vi "GetNI_SynthFocus_25.vi"(0 "Digitizer Settings":T4={"Digitizer delay (us) "=0.0, "rf points per line"=2048, "lines per plane"=128, "Samp Rate (Hz)"=100000000.0, "Additional dig delay (us)"=0.0, "Voltage Scale"=0.4, "Pre-Looks"=0, "Offset delay (us)"=0.0, "bits A/D"=8, "Avg Num"=1, "DigTimeOut"=5.0, "Rel Dig Delay"=0.0, "Dig Ch"=0, "LeCroyCluster"={"LeCroy Channels"=[TRUE, FALSE, FALSE, FALSE], "LC read pt offset"=0.0, "Sweep Avg"=FALSE}, "Main Digitizer"=enum."NI Digitizer", "Dig Config"=enum."Single channel", "Digitizer ID Cluster"={"Acqiris/Alazar/SP ID"=[], "NI Instr Handles"=[], "LeCroy VISA"="", "GaGe Handle"={"Handle"=0, "Sample size"=0, "Resolution"=0, "Offset"=0, "Channels"=0, "Boards"=0}, "ATS Ref"="ATS9350", "Acqiris Address"=["PCI::INSTR0"], "ADQRef"=refnum, "adq_cu_ptr"=refnum}, "Trigger Settings"={"Trig Source"=1, "Trig Coupling"=0, "Trig Slope"=0, "Level (mV)"=1500.0}, "Bulk Acq"=FALSE, "Bulk Start Indexes"=[], "Data Ref RF"=refnum, "NI ID/Channel"=[], "Total Dig CH"=1, "Xtra Ann Trig delay (us)"=10.0, "Fix Z Delay?"=FALSE, "One Way Transmission?"=FALSE, "Data Ref Log"=refnum} {"Trigger Settings"."Trig Slope" items=["Positive", "Negative"]; "Trigger Settings"."Level (mV)" format="%.2f"; "Trigger Settings"."Trig Coupling" items=["DC 1 MOhm", "AC 1 MOhm", "DC 50 Ohm", "AC 50 Ohm"]; "Trigger Settings"."Trig Source" items=["Chan 1", "External"]; "Rel Dig Delay" format="%.2f"; "DigTimeOut" format="%.2f"; "Avg Num" min=1; "Offset delay (us)" format="%.2f"; "Additional dig delay (us)" format="%.2f"; "Digitizer delay (us)" format="%.2f"}, 7 "errorin":errorcluster, 8 "File Array":string[](array[string]), 9 "Ann Array Params":T1={"Synth Foc?"=FALSE, "Focal Zones"=41, "Switch T/R"=0, "Trans Geometry (mm)"={"Transducer"=0, "Geo Focus"=12.0, "a (radius)"=3.0, "# of rings"=5, "kerf space "=0.1, "Center Freq"=12.0}, "Sub Ap Excite?"=FALSE, "Full Array Scan?"=FALSE, "Xmt/Rcv"={"XMIT"=[TRUE, TRUE, TRUE, TRUE, TRUE], "RCV"=[TRUE, TRUE, TRUE, TRUE, TRUE]}, "PulseSpacing (us)"=0.0, "Xmit Ring"=0, "XMIT CHS"=0, "RCV CHS"=0, "GPU?"=FALSE, "Save TIFF?"=FALSE, "downfactor"=1, "RCV 1CH"=0} {"RCV 1CH" items=["All", "1", "2", "3", "4", "5"]; "Trans Geometry (mm)"."Transducer" items=["6D 12R 40 MHz"=0, "10D 31R 20 MHz"=1, "10D 23R 20 MHz"=2, "6D 23R 40 MHz"=3, "4.5D 10.7R 40 MHz"=4, "9D 23.5R 20 MHz"=5, "9D 25.8R 20MHz"=6, "Enter"=99]; "Switch T/R" min=1 max=5 step=1}, 10 "lines per plane":i32, 15 "Reverse?":bool) -> (17 "Raw VGain (scale)":dbl, 18 "Gain Array":T8(array[cluster]), 21 "VGain (dB)":dbl, 27 "error out":errorcluster)   [LabVIEW 2022 SP3]
uses:
  -DigitizerRoutines/DigitizerSettings.ctl
  -DigitizerRoutines/Digitizer.ctl
  -DigitizerRoutines/DigConfig.ctl
  -DigitizerRoutines/DigitizerID.ctl
  C:/Windows/System32/ADQAPI_dotNet_helper.dll
  Annular Array/-AnnularRoutines/AnnularArray.ctl
  Annular Array/-AnnularRoutines/TransGeometry.ctl
  Annular Array/-AnnularRoutines/ArrayGeometry.ctl
  <instrlib>/niScope/Acquire/Fetch/niScope Multi Fetch Binary 8.vi
  Motion Controllers/-MotionRoutines/MotionGlobals.vi
  Annular Array/-SynthApperture/ProcImageHD_I16.vi
panel:
  out "read time":u32
  out "synth foc time":u32
  out "Numeric":i32
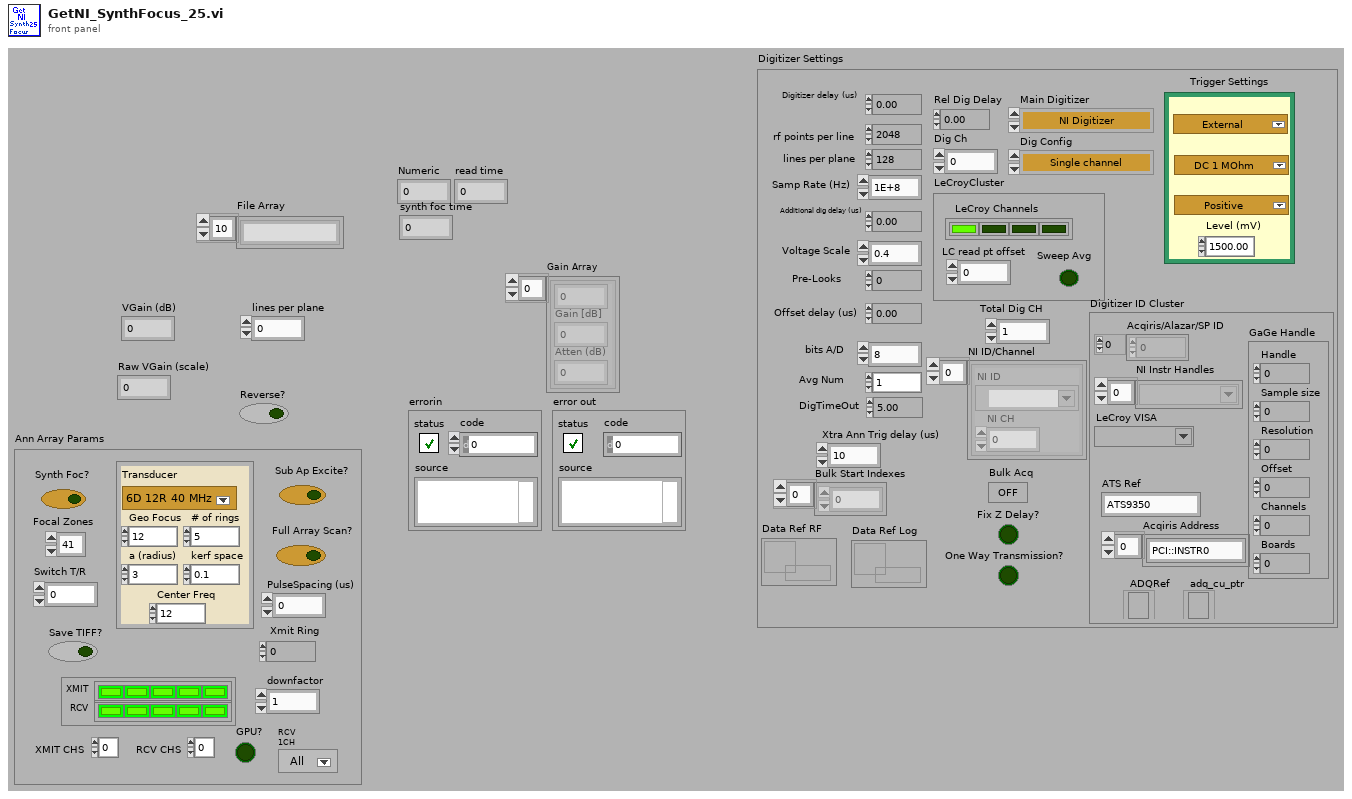
[diagram p1: front panel]
types:
  T1 = typedef "AnnularArray.ctl" = cluster{"Synth Foc?":bool, "Focal Zones":i16, "Switch T/R":i16, "Trans Geometry (mm)":T2, "Sub Ap Excite?":bool, "Full Array Scan?":bool, "Xmt/Rcv":cluster{"XMIT":bool[], "RCV":bool[]}, "PulseSpacing (us)":sgl, "Xmit Ring":i32, "XMIT CHS":u8, "RCV CHS":u8, "GPU?":bool, "Save TIFF?":bool, "downfactor":i32, "RCV 1CH":u16}
  T2 = typedef "TransGeometry.ctl" = cluster{"Transducer":T3, "Geo Focus":dbl, "a (radius)":dbl, "# of rings":i32, "kerf space ":dbl, "Center Freq":dbl}
  T3 = typedef "ArrayGeometry.ctl" = u16
  T4 = typedef "DigitizerSettings.ctl" = cluster{"Digitizer delay (us) ":dbl, "rf points per line":i32, "lines per plane":i32, "Samp Rate (Hz)":dbl, "Additional dig delay (us)":dbl, "Voltage Scale":dbl, "Pre-Looks":i32, "Offset delay (us)":dbl, "bits A/D":i8, "Avg Num":i32, "DigTimeOut":sgl, "Rel Dig Delay":sgl, "Dig Ch":i32, "LeCroyCluster":cluster{"LeCroy Channels":bool[], "LC read pt offset":dbl, "Sweep Avg":bool}, "Main Digitizer":T5, "Dig Config":T6, "Digitizer ID Cluster":T7, "Trigger Settings":cluster{"Trig Source":u16, "Trig Coupling":u16, "Trig Slope":u16, "Level (mV)":dbl}, "Bulk Acq":bool, "Bulk Start Indexes":i32[], "Data Ref RF":refnum<data-value>, "NI ID/Channel":cluster{"NI ID":refnum<k15>, "NI CH":i32}[], "Total Dig CH":i32, "Xtra Ann Trig delay (us)":dbl, "Fix Z Delay?":bool, "One Way Transmission?":bool, "Data Ref Log":refnum<data-value>}
  T5 = typedef "Digitizer.ctl" = enum16{"Acqiris Digitizer", "NI Digitizer", "LeCroy", "GaGe", "AlazarTech", "No Digitizer", "Teledyne"}
  T6 = typedef "DigConfig.ctl" = enum16{"Single channel", "2 Chans w/ 2 Acqiris", "2 Chans w/ 1 Acqiris", "5-CH Pulser New", "5-CH pulser w/ ann array", "5-pass style ann array", "Empty"}
  T7 = typedef "DigitizerID.ctl" = cluster{"Acqiris/Alazar/SP ID":u32[], "NI Instr Handles":refnum<k15>[], "LeCroy VISA":refnum<visa-resource-name>, "GaGe Handle":cluster{"Handle":u32, "Sample size":u32, "Resolution":i32, "Offset":i32, "Channels":u32, "Boards":u32}, "ATS Ref":string, "Acqiris Address":string[], "ADQRef":refnum<k24>, "adq_cu_ptr":refnum<k24>}
  T8 = cluster{sgl, "Gain [dB]  ":sgl, "Atten (dB)":sgl}[]
  T9 = cluster{"actualSamples":i32, "absoluteInitialX":dbl, "relativeInitialX":dbl, "xIncrement":dbl, "offset":dbl, "gain":dbl, "reserved1":dbl, "reserved2":dbl}[]
  T10 = cluster{"actualSamples":i32, "absoluteInitialX":dbl, "relativeInitialX":dbl, "xIncrement":dbl, "offset":dbl, "gain":dbl, "reserved1":dbl, "reserved2":dbl}
  T11 = cluster{"low cutoff":i32, "order":i32, "high cutoff":i32}
  T12 = cluster{"FIR Windowed Coefficients":dbl[], "Filter Prams":cluster{"low cutoff":i32, "order":i32, "high cutoff":i32}}
  T13 = cluster{sgl, "Gain [dB]  ":sgl, "Atten (dB)":sgl}
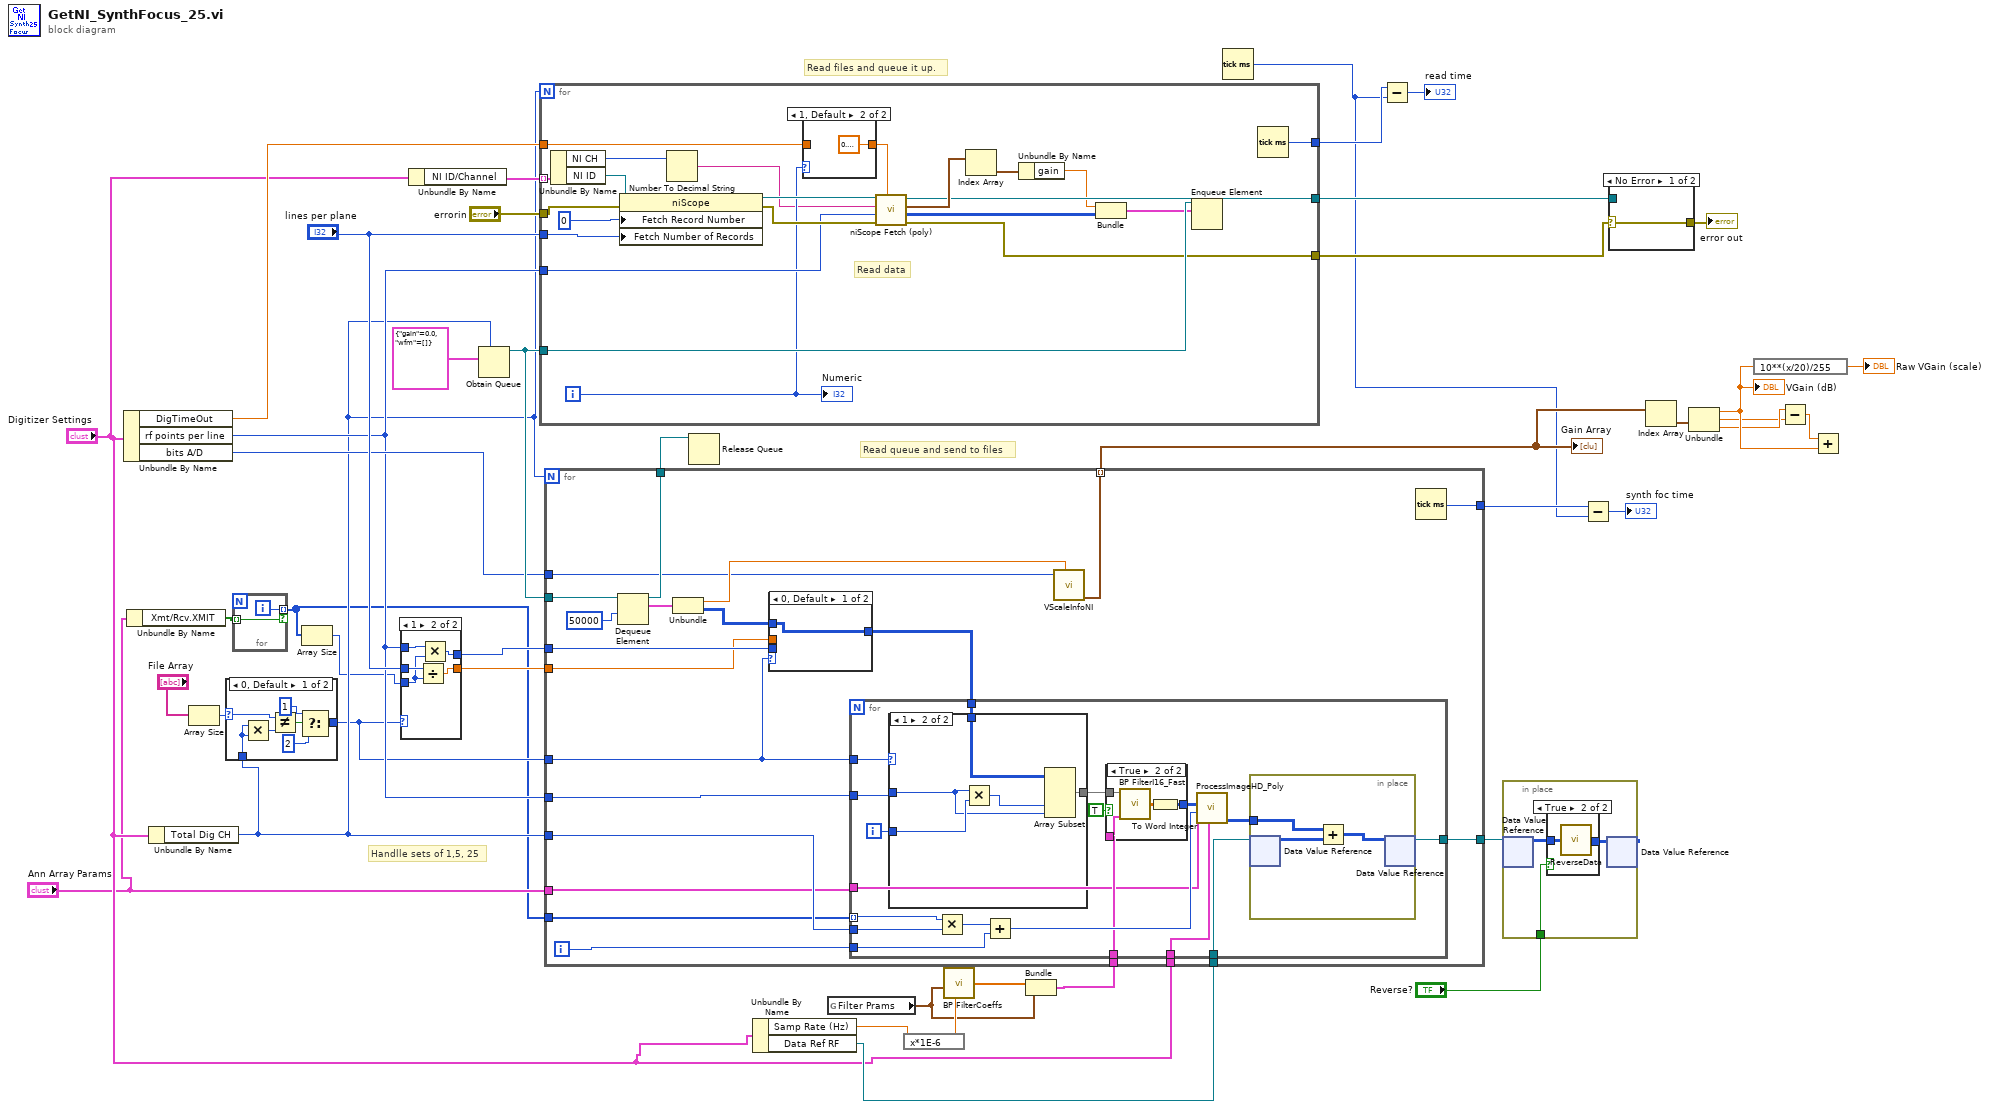
[diagram p0: block diagram]
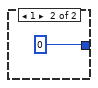
[diagram p3: hidden frame]
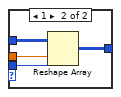
[diagram p5: hidden frame]
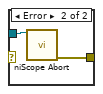
[diagram p8: hidden frame]
diagram:
  # "Handlle sets of 1,5, 25"
  # "Read files and queue it up."
  # "Read queue and send to files"
  n1 = Unbundle By Name("Digitizer Settings") -> ("DigTimeOut"=w13:sgl, "rf points per line"=w14:i32, "bits A/D"=w15:i8)
  n2 = Unbundle By Name("Ann Array Params") -> ("Xmt/Rcv.XMIT"=w4:bool[])
  n3 = Unbundle By Name("Digitizer Settings") -> ("Total Dig CH"=w9:i32)
  n4 = Array Size(array="File Array") -> (size(s)=w8:i32)
  n5 = case shown="0, Default" w8 {
    selector: w8 -> [w50 _]
    tunnel: w9 -> [w49 _]
    tunnel: [w48 0] -> w7
    frame 0, Default {
      n6 = Multiply(x=w49, y=w49) -> (x*y=w46:i32)
      n7 = Not Equal?(x=w50, y=w46) -> (x != y?=w47:bool)
      n8 = Select(t=1, s=w47, f=2) -> (s? t:f=w48:i32)
    }
    frame 1 {
    }
  }
  n9 = for {
    tunnel: w4 -> [w53] mode=indexing
    tunnel: [w52] -> w1 mode=indexing if=w53
    i -> [w52]
  }
  n10 = Array Size(array=w1) -> (size(s)=w2:i32)
  n11 = case shown="1" w7 {
    tunnel: [w55 w59] -> w23
    tunnel: w14 -> [w55 w58]
    tunnel: [w54 w60] -> w22
    tunnel: "lines per plane" -> [w54 w57]
    tunnel: w2 -> [_ w56]
    frame 0, Default {
    }
    frame 1 {
      n12 = Divide(x=w57, y=w56) -> (x/y=w60:dbl)
      n13 = Multiply(x=w58, y=w56) -> (x*y=w59:i32)
    }
  }
  n14 = Unbundle By Name("Digitizer Settings") -> ("NI ID/Channel"=w11:cluster{"NI ID":refnum<k15>, "NI CH":i32}[])
  n15 = Obtain Queue(max queue size (-1, unlimited)=w9, element data type=cluster{"gain":dbl, "wfm":i8[][]} {"gain"=0.0, "wfm"=[]}) -> (queue out=w32:refnum<queue>)  [unwired: 3 in, 2 out]
  n16 = for {
    N: w9 -> [_]
    tunnel: w13 -> [w66]
    tunnel: w14 -> [w74]
    tunnel: "errorin" -> [w82]
    tunnel: "lines per plane" -> [w77]
    tunnel: [w76] -> w41
    tunnel: w32 -> [w73]
    tunnel: [w69] -> w31
    tunnel: [w68] -> w30
    tunnel: w11 -> [w64] mode=indexing
    i -> [w67]
    # "Read data"
    n17 = Unbundle By Name(w64) -> ("NI CH"=w62:i32, "NI ID"=w63:refnum<k15>)
    n18 = property class="niScope"(reference=w63, error in=w82, "Fetch Record Number"=0, "Fetch Number of Records"=w77) -> (reference out=w75:refnum<k15>, error out=w81:errorcluster)
    n19 = Number To Decimal String(number=w62) -> (decimal integer string=w61:string)  [unwired: 1 in]
    n20 = case shown="1, Default" w67 {
      tunnel: w66 -> [w83 _]
      tunnel: [w83 sgl 0.1 ("DigTimeOut")] -> w65
      frame 0 {
      }
      frame 1, Default {
      }
    }
    n21 = call-poly <instrlib>:"niScope Fetch (poly).vi"("timeout"=w65, "error in"=w81, "numSamples"=w74, "channels"=w61, "instrument handle"=w75) -> ("error out"=w69:errorcluster, "wfm"=w71:i8[][], "wfm info"=w80:T9, "instrument handle out"=w76:refnum<k15>)  [unwired: 3 out]
    n22 = Index Array(array=w80) -> (element=w79:T10)  [unwired: 1 in]
    n23 = Unbundle By Name(w79) -> ("gain"=w72:dbl)
    n24 = Bundle("gain"=w72, "wfm"=w71) -> (w70:cluster{"gain":dbl, "wfm":i8[][]})  [unwired: 1 in]
    n25 = Enqueue Element(queue=w73, element=w70) -> ()  [unwired: 2 in, 3 out]
    n26 = Tick Count (ms)() -> (millisecond timer value=w68:u32)
    "Numeric" <- w67
  }
  n27 = Unbundle By Name("Digitizer Settings") -> ("Samp Rate (Hz)"=w16:dbl, "Data Ref RF"=w12:refnum<data-value>)
  n28 = global read "MotionGlobals.vi" "Filter Prams"() -> (w17:T11)
  n29 = expression code="x*1E-6"(w16) -> (w18:dbl)
  n30 = call "BP FilterCoeffs.vi"("sample rate MHz"=w18, "Filter Prams"=w17) -> ("FIR Windowed Coefficients"=w19:dbl[])  [unwired: 4 in]
  n31 = Bundle("FIR Windowed Coefficients"=w19, "Filter Prams"=w17) -> (w20:T12)  [unwired: 1 in]
  n32 = for {
    N: w9 -> [_]
    tunnel: w23 -> [w106]
    tunnel: w14 -> [w105]
    tunnel: w22 -> [w98]
    tunnel: [w104] -> w33 mode=indexing
    tunnel: w32 -> [w103]
    tunnel: [w97] -> w25
    tunnel: [w96] -> w29
    tunnel: w7 -> [w95]
    tunnel: w12 -> [w94]
    tunnel: w9 -> [w88]
    tunnel: w20 -> [w91]
    tunnel: w15 -> [w90]
    tunnel: "Digitizer Settings" -> [w89]
    tunnel: "Ann Array Params" -> [w87]
    tunnel: [w86] -> w5
    tunnel: w1 -> [w85]
    i -> [w93]
    n33 = Dequeue Element(queue=w103, timeout in ms (-1)=50000) -> (queue out=w97:refnum<queue>, element=w102:cluster{"gain":dbl, "wfm":i8[][]})  [unwired: 1 in, 2 out]
    n34 = Unbundle(w102) -> ("gain"=w101:dbl, "wfm"=w100:i8[][])
    n35 = case shown="0, Default" w95 {
      tunnel: w106 -> [_ w111]
      tunnel: w100 -> [w107 w110]
      tunnel: [w107 w109] -> w92
      tunnel: w98 -> [_ w108]
      frame 0, Default {
      }
      frame 1 {
        n36 = Reshape Array(w110, w108, w111) -> (w109:i8[][])
      }
    }
    n37 = for {
      tunnel: w105 -> [w129]
      tunnel: w92 -> [w128]
      tunnel: w95 -> [w127]
      tunnel: w93 -> [w124]
      tunnel: w94 -> [w121]
      tunnel: w91 -> [w118]
      tunnel: w89 -> [w116]
      tunnel: w88 -> [w115]
      tunnel: w87 -> [w114]
      tunnel: [w113] -> w86
      tunnel: w85 -> [w112] mode=indexing
      i -> [w126]
      n38 = case shown="1" w127 {
        tunnel: [w138 w139] -> w120
        tunnel: w126 -> [_ w143]
        tunnel: w129 -> [_ w141]
        tunnel: w128 -> [w138 w140]
        frame 0, Default {
        }
        frame 1 {
          n39 = Multiply(x=w141, y=w143) -> (x*y=w142:i32)
          n40 = Array Subset(array=w140, index (col)=w142, length (col)=w141) -> (w139:i8[][])  [unwired: 2 in]
        }
      }
      n41 = Multiply(x=w112, y=w115) -> (x*y=w125:i32)
      n42 = Add(x=w125, y=w124) -> (x+y=w123:i32)
      n43 = case shown="True" TRUE {
        tunnel: w120 -> [w130 w133]
        tunnel: [w130 w132] -> w119
        tunnel: w118 -> [_ w131]
        frame False {
        }
        frame True {
          n44 = call "BP FilterI16_Fast.vi"("Filter"=w131, "Array in"=w133) -> ("Filtered X"=w134:dbl[][])  [unwired: 4 in]
          n45 = To Word Integer(number=w134) -> (16bit integer=w132:i16[][])
        }
      }
      n46 = call-poly "ProcessImageHD_Poly.vi"("Digitizer Settings"=w116, "Ann Array Params"=w114, "T/R Ring"=w123, "Scan Data In"=w119) -> ("Synth App Out"=w122:i16[][])  [unwired: 4 in, 1 out]
      n47 = in-place {
        in-place-border: w122 -> [w136]
        n48 = in-place-dvr #1(w121) -> (w135:i16[][])  [unwired: 1 out]
        n49 = Add(x=w136, y=w135) -> (x+y=w137:i16[][])
        n50 = in-place-dvr #1(w137) -> (w113:refnum<data-value>)  [unwired: 1 out]
      }
    }
    n51 = call "VScaleInfoNI.vi"("A/D bits"=w90, "gain"=w101) -> ("Voltage Scale"=w104:T13)  [unwired: 5 in, 3 out]
    n52 = Tick Count (ms)() -> (millisecond timer value=w96:u32)
  }
  "Gain Array" <- w33
  n53 = Release Queue(queue=w25) -> ()  [unwired: 2 in, 3 out]
  n54 = Tick Count (ms)() -> (millisecond timer value=w28:u32)
  n55 = Subtract(x=w30, y=w28) -> (x-y=→"read time":u32)
  n56 = in-place {
    in-place-border: "Reverse?" -> [w144]
    n57 = in-place-dvr #2(w5) -> (w146:i16[][])  [unwired: 1 out]
    n58 = case shown="True" w144 {
      tunnel: w146 -> [w147 w149]
      tunnel: [w147 w148] -> w145
      frame False {
      }
      frame True {
        n59 = call "ReverseData.vi"("Array in"=w149) -> ("Array out"=w148:i16[][])
      }
    }
    n60 = in-place-dvr #2(w145) -> ()  [unwired: 2 out]
  }
  n61 = Subtract(x=w29, y=w28) -> (x-y=→"synth foc time":u32)
  n62 = case shown="No Error" w31 {
    selector: w31 -> [w150 _]
    tunnel: w41 -> [_ w152]
    tunnel: [w150 w151] -> w42
    frame No Error {
    }
    frame Error {
      n63 = call <instrlib>:"niScope Abort.vi"("instrument handle"=w152) -> ("error out"=w151:errorcluster)  [unwired: 1 in, 13 out]
    }
  }
  "error out" <- w42
  n64 = Index Array(array=w33) -> (element=w40:T13)  [unwired: 1 in]
  n65 = Unbundle(w40) -> (w39:sgl, "Gain [dB]"=w37:sgl, "Atten (dB)"=w38:sgl)
  "VGain (dB)" <- w39
  n66 = expression code="10**(x/20)/255"(w39) -> (→"Raw VGain (scale)":sgl)
  n67 = Subtract(x=w38, y=w37) -> (x-y=w36:sgl)
  n68 = Add(x=w36, y=w39) -> ()  [unwired: 1 out]
